vi "NR_crc24a.vi"(0 "appended path":path, 5 "LDPC_base_graph":dbl, 7 "i_ls":dbl, 11 "error in (no error)":errorcluster caption="错误输入（无错误）", 12 "info_data":dbl[](array[numeric])) -> (3 "C":dbl, 4 "Zc":dbl, 6 "F":dbl, 10 "cdblkseg_data":dbl[][](array[numeric]), 15 "error out":errorcluster caption="错误输出")   [LabVIEW 2015]
panel:
  out "K_p":dbl
  out "K":dbl
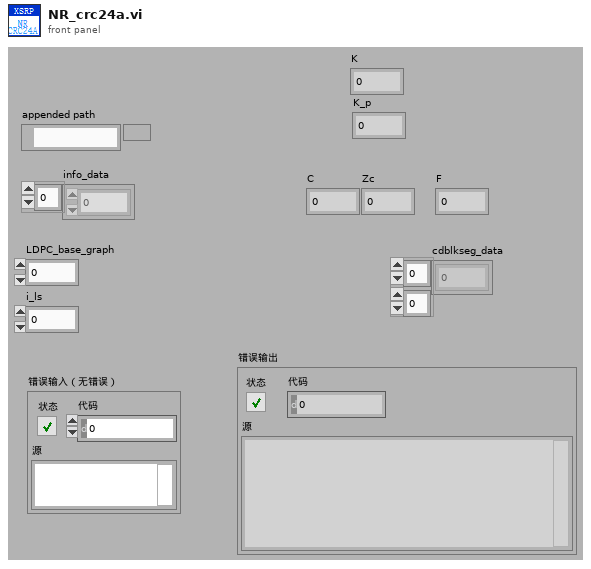
[diagram p1: front panel]
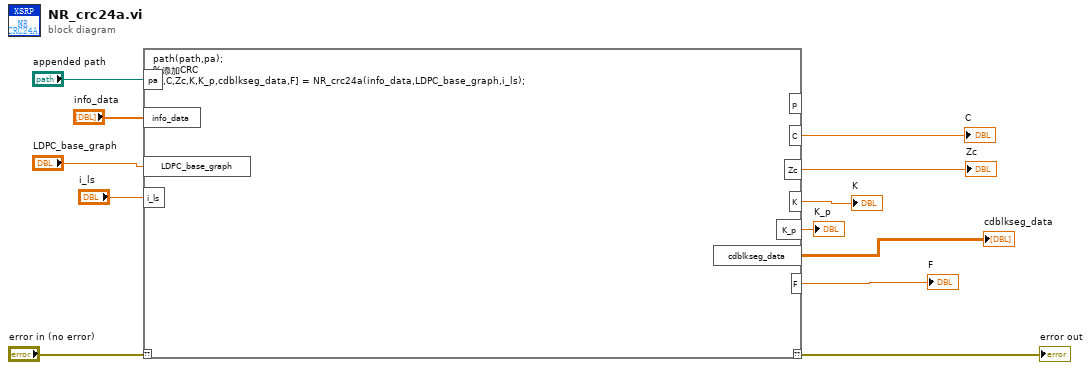
[diagram p0: block diagram]
diagram:
  n1 = script code="path(path,pa);\n%添加CRC\n[p,C,Zc,K,K_p,cdblkseg_data,F] = NR_crc24a(info_data,LDPC_base_graph,i_ls);"("??"="error in (no error)", "pa"="appended path", "info_data"="info_data", "LDPC_base_graph"="LDPC_base_graph", "i_ls"="i_ls") -> ("??"=→"error out":errorcluster, "C"=→"C":dbl, "Zc"=→"Zc":dbl, "K"=→"K":dbl, "K_p"=→"K_p":dbl, "F"=→"F":dbl, "cdblkseg_data"=→"cdblkseg_data":dbl[][])  [unwired: 1 out]
